vi "Moisture_SW_Update.vi"(0 "State":enum16{"Stop", "Continue", "Update"}(ring)=enum."Update", 5 "Average":dbl, 7 "Delta":dbl, 11 "Error In":errorcluster) -> (15 "Error Out":errorcluster)   [LabVIEW 2014]
uses:
  type defs/moisture_SW_control.ctl
panel:
  in  "Dither Values":dbl[](array[numeric])
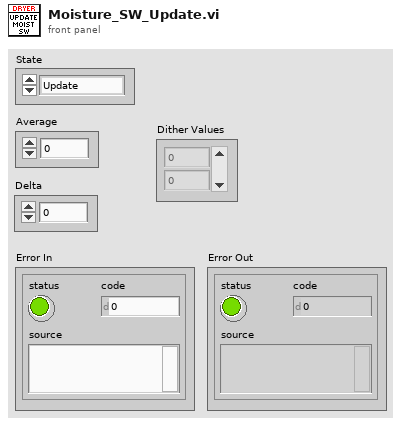
[diagram p1: front panel]
types:
  T1 = typedef "moisture_SW_control.ctl" = cluster{"State":enum16{"Stop", "Continue", "Update"}, "Data":variant}
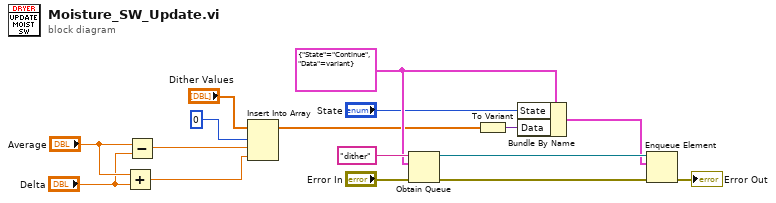
[diagram p0: block diagram]
diagram:
  w13 = T1 {"State"=enum."Continue", "Data"=variant}
  n1 = Add(x="Average", y="Delta") -> (x+y=w2:dbl)
  n2 = Subtract(x="Average", y="Delta") -> (x-y=w3:dbl)
  n3 = Insert Into Array(array="Dither Values", index=0, new element #1=w3, new element #2=w2) -> (w1:dbl[])
  n4 = Obtain Queue(name (unnamed)="dither", element data type=w13, error in (no error)="Error In") -> (queue out=w15:refnum<queue>, error out=w14:errorcluster)  [unwired: 2 in, 1 out]
  n5 = To Variant(anything=w1) -> (Variant=w11:variant)
  n6 = Bundle By Name(cluster=w13, "State"="State", "Data"=w11) -> (w10:T1)
  n7 = Enqueue Element(queue=w15, element=w10, error in (no error)=w14) -> (error out=→"Error Out":errorcluster)  [unwired: 1 in, 2 out]
